vi "Write Data to File.vi"(8 "error in (no error)":errorcluster, 10 "Data In":string, 11 "File in":refnum<file>) -> (0 "error out":errorcluster, 3 "File out":refnum<file>)   [LabVIEW 2017]
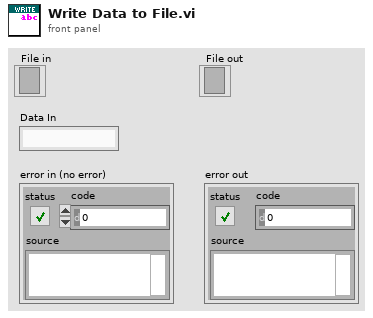
[diagram p1: front panel]
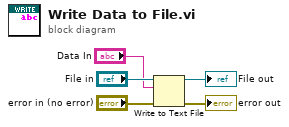
[diagram p0: block diagram]
diagram:
  n1 = Write to Text File(file (use dialog)="File in", text="Data In", error in="error in (no error)") -> (refnum out=→"File out":refnum<file>, error out=→"error out":errorcluster)  [unwired: 2 out]
